vi "Write Components.vi"(8 "error in (no error)":errorcluster, 10 "Components":refnum<class "1553 Component.lvclass">[](array[class]), 11 "1553 Board in":refnum<class "1553 Session.lvclass">) -> (0 "error out":errorcluster, 3 "1553 Board out":refnum<class "1553 Session.lvclass">)   [LabVIEW 2020, in "BCI-1553 API.lvlib" / "1553 Session.lvclass"]
doc: "Write accessor for 1553 Session Components. Depending on Session configuration, there may be up to 8 Components in a 1553 Session. Do not use this accessor to perform 1553 Session initialization. This accessor should only be used when a Read Components call was done previously to retrieve existing 1553 Session Components."
uses:
  1553 Session.lvclass
  1553 Component/1553 Component.lvclass
  1553 Session.lvclass/1553 Session.ctl
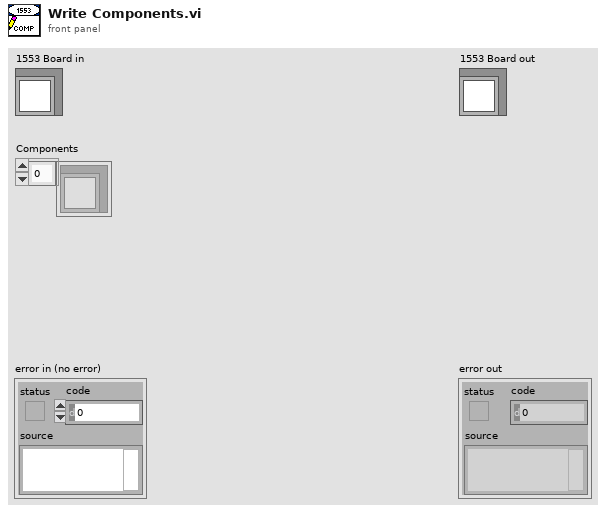
[diagram p1: front panel]
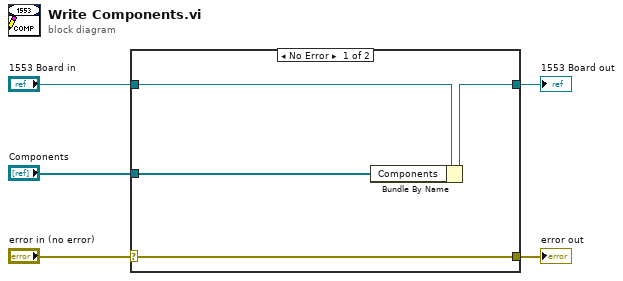
[diagram p0: block diagram]
diagram:
  n1 = case shown="No Error" "error in (no error)" {
    selector: "error in (no error)" -> [w9 w11]
    tunnel: [w9 w11] -> w4
    tunnel: [w7 w10] -> w2
    tunnel: "1553 Board in" -> [w8 w10]
    tunnel: "Components" -> [w6 _]
    frame No Error {
      n2 = Bundle By Name(cluster=w8, "Components"=w6) -> (w7:refnum<class "1553 Session.lvclass">)
    }
    frame Error {
    }
  }
  "error out" <- w4
  "1553 Board out" <- w2
